vi "GUID Lookup.vi"() -> ()   [LabVIEW 2015, in "Protection and Counter Addon Shared.lvlib"]
doc: "Use this Global VI to access the GUIDs assigned to the page resources of the Custom Device."
uses:
  Protection and Counter Addon Shared.lvlib
panel:
  in  "Tab Control":enum32{"GUIDS", "Constants"}(tab)
  in  "Protection Valid GUID":string="4d205a57-60cc-4efa-a0ca-6814bbbf829a"
  in  "Counter Valid GUID":string="afb8a5df-af0a-415b-a4a9-80e19e724a73"
  in  "Custom Device GUID":string="4d3156ae-de1b-463a-a86e-31c1bc069b17"
  in  "Frame Configuration GUID":string="bc0c6957-d4ef-4e45-aa02-83c9b233598c"
  in  "Protection Value GUID":string="ed369b01-8bb7-4d5d-8463-e4aaa20f9c2b"
  in  "Counter Value GUID":string="94e87467-031b-484c-a85e-bcbac581524d"
  in  "Custom Device GUID_Disabled":string="ac3d5221-c9c0-44f4-a291-06920e8a9c9a"
  in  "Enable Disable GUID":string="4733d1e7-fc02-4e27-be4e-9d2e12f6fe6f"
  in  "Protection Valid Channel GUID":string="fd6a7400-7849-4da5-96c3-5ff30bdc4abb"
  in  "Status GUID":string="9ef2cd96-dffa-48ea-ae2c-932b4b88a115"
  in  "Status Channel GUID":string="6d842445-75a9-45cc-a4de-fe1217a46de2"
  in  "Outgoing Page GUID":string="ac3e6a25-b54a-448b-bc03-298d2e8e37c0"
  in  "Outgoing Event Page GUID":string="f7870371-b1e4-4bce-a037-eb1b5f7e56a7"
  in  "Outgoing Cyclic GUID":string="a83bc0a9-6c38-418b-b0b7-47e877787b3f"
  in  "Outgoing Frame Page GUID":string="2db218fe-96df-4f04-8b61-900a312ea43d"
  in  "Incoming Page GUID":string="ecc25de3-c2ab-46d7-9bc3-042f52653143"
  in  "Incoming Single Point Page GUID":string="45d997b9-be87-4536-8aa7-486032a53b20"
  in  "Incoming Frame Page GUID":string="b05244b8-7523-4075-97f9-80c23ea41b5d"
  in  "Signal Page GUID":string="4b95dee7-8d64-48ce-932c-f5fdd14e4d4c"
  in  "Receive Time GUID":string="03ef744a-f736-4cb8-9a6d-2a50c922df62"
  in  "Time Difference GUID":string="e7dc4b72-c845-404c-9a5f-2435f1763b64"
  in  "Information Page GUID":string="bad551ee-44df-483f-8901-46140a12e346"
  in  "Outgoing Cyclic Event GUID":string="8bdca9b3-9695-43a6-96c0-38fee5afce4b"
  in  "Protection Valid Name":string="Protection Valid"
  in  "Counter Valid Name":string="Counter Valid"
  in  "Frame.Disable":string="Frame.Disable"
  in  "Frame.Trigger":string="Frame.Trigger"
  in  "Status Page Name":string="Status"
  in  "Frame Configuration Page Name":string="Frame Configuration"
  in  "Frame Configuration":string="Frame Configuration Settings"
  in  "Protection Value":string="Protection"
  in  "Protection Valid Channel Page Name":string="Valid"
  in  "Frame.Transmit Trigger":string="Transmit Trigger"
  in  "Frame.Disable Transmission":string="Disable Transmission"
  in  "Status.Period":string="Period"
  in  "Status.ErrorStatus":string="Error Status"
  in  "Status.Duration":string="Duration"
  in  "XNET.Database":string="XNET.Database"
  in  "XNET.Cluster":string="XNET.Cluster"
  in  "XNET.Port":string="XNET.Port"
  in  "XNET.Rate":string="XNET.Rate"
  in  "XNET.Termination":string="XNET.Termination"
  in  "XNET.FDRate":string="XNET.FDRate"
  in  "XNET.IOMode":string="XNET.IOMode"
  in  "OnCompileSettings":string="OnCompileSettings"
  in  "SignalsRef":string="SignalsRef"
  in  "ProtectionsAndCountersRefs":string="ProtectionAndCountersRefs"
  in  "StatusRefs":string="StatusRefs"
  in  "XNET.LoopPriority":string="XNET.LoopPriority"
  in  "XNET.Legacy":string="XNET.Legacy"
  in  "Outgoing Page Name":string="Outgoing"
  in  "Outgoing Event Page Name":string="Event Triggered"
  in  "Outgoing Cyclic Name":string="Cyclic"
  in  "Incoming Page Name":string="Incoming"
  in  "Incoming Single Point Page Name":string="Single Point"
  in  "Frame.ID":string="ID"
  in  "Bitfile 986x":string="Bitfile 986x"
  in  "Receive Time Name":string="Receive Time"
  in  "Time Difference Name":string="Time Difference"
  in  "Information Name":string="Frame Information"
  in  "RIO Device 986x":string="RIO Device 986x"
  in  "Enable 986x":string="Enable 986x"
  in  "RT Bitfile Location":path=path "c:/ni-rt/NIVeriStand/XNET"
  in  "Outgoing Cyclic Event Name":string="Cyclic Event"
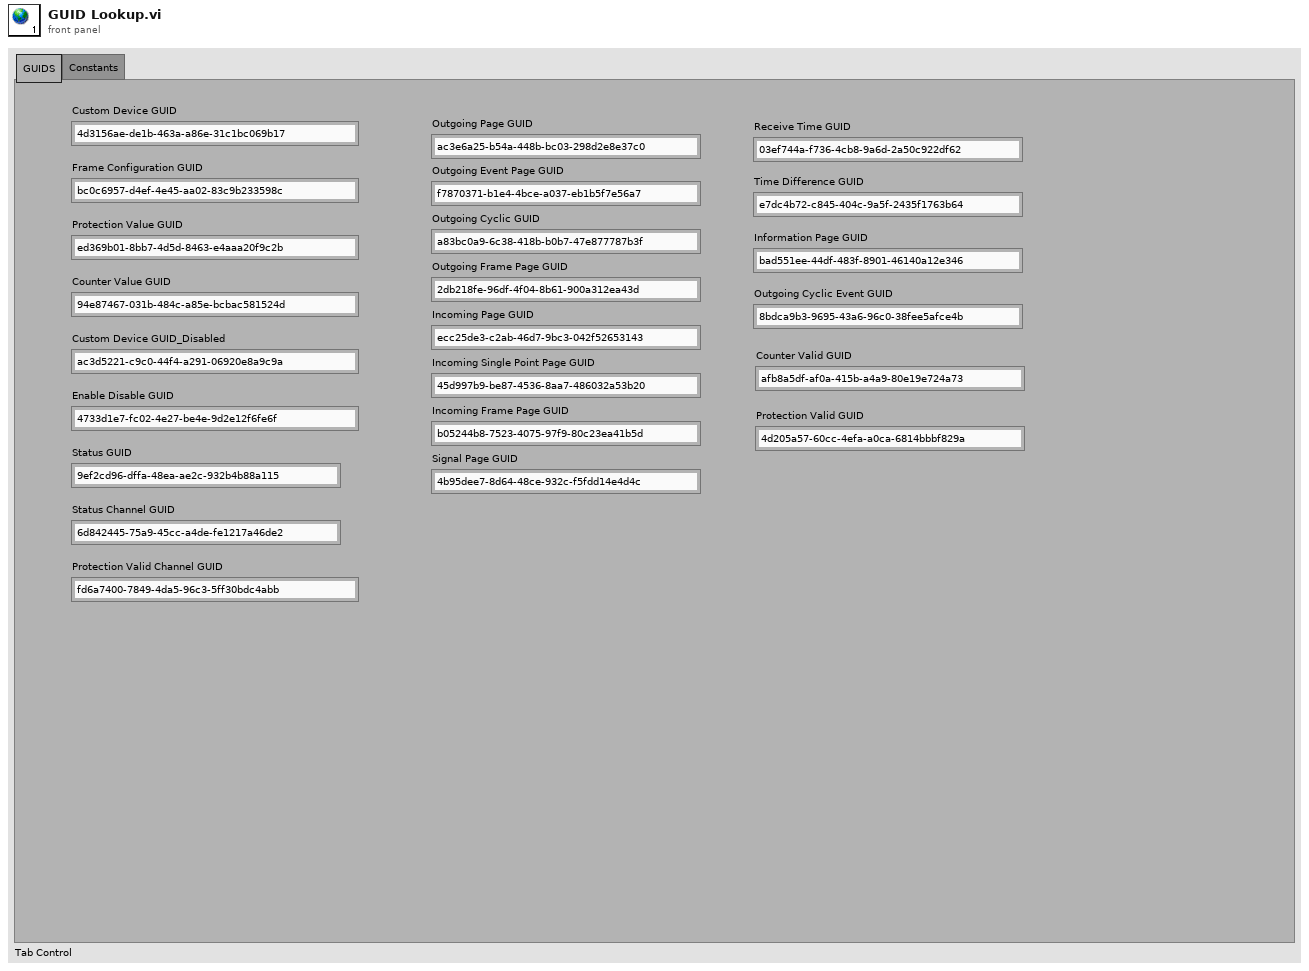
[diagram p1: front panel]
diagram:
